vi "About.vi"(10 "窗口边界":T1) -> ()   [LabVIEW 2015]
doc: "本VI是为《我和LabVIEW》一书编写的示例。\n关于本书的介绍请参考网页：\nhttp://ruanqizhen.spaces.live.com/blog/cns!5852D4F797C53FB6!4310.entry"
uses:
  <vilib>/Utility/miscctls.llb/LVRectTypeDef.ctl
  user32.dll
panel:
  # "上海华湘计算机通讯工程有限公司\nShanghai Huaxiang \nCommunication Engineering Co.,Ltd.\n\nSwitch Matrix\nV1.0"
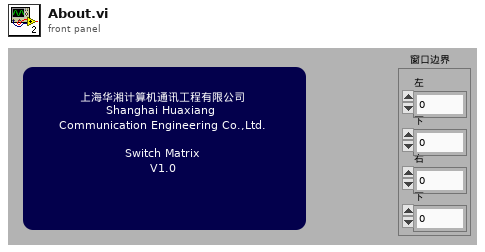
[diagram p1: front panel]
types:
  T1 = typedef "LVRectTypeDef.ctl" = cluster{"Left":i16, "Top":i16, "Right":i16, "Bottom":i16}
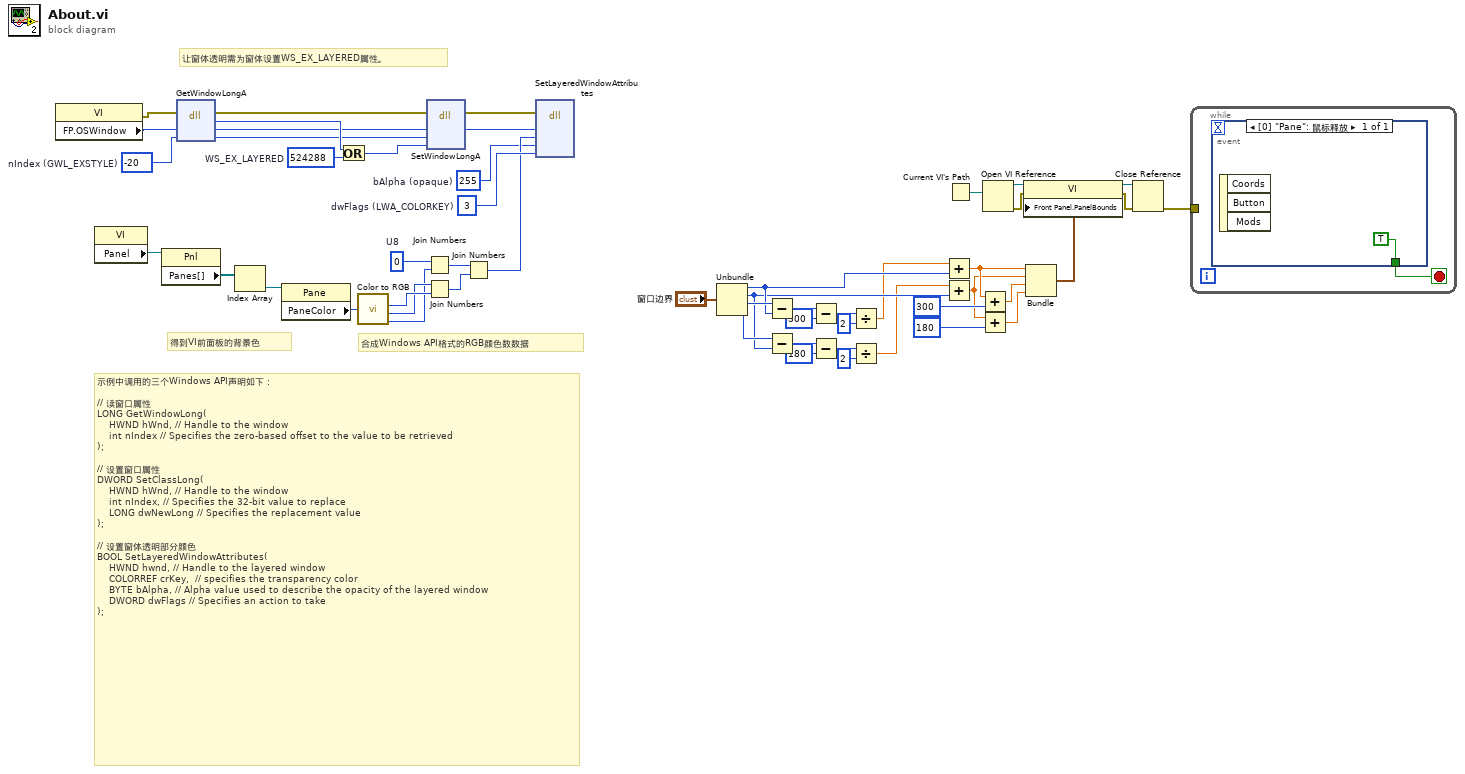
[diagram p0: block diagram]
diagram:
  w41 = 524288  # WS_EX_LAYERED
  w38 = -20  # nIndex (GWL_EXSTYLE)
  w44 = 255  # bAlpha (opaque)
  w45 = u8 0  # U8
  w49 = 3  # dwFlags (LWA_COLORKEY)
  # "示例中调用的三个Windows API声明如下：\n\n// 读窗口属性\nLONG GetWindowLong(      \n    HWND hWnd,\t// Handle to the window\n    int nIndex\t// Specifies the zero-based offset to the value to be retrieved\n);\n\n// 设置窗口属性\nDWORD SetClassLong(      \n    HWND hWnd,\t// Handle to the window\n    int nIndex,\t// Specifies the 32-bit value to replace\n    LONG dwNewLong // Specifies the replacement value\n);\n\n// 设置窗体透明部分颜色\nBOOL SetLayeredWindowAttributes(      \n    HWND hwnd,\t// Handle to the layered window\n    COLORREF crKey,  // specifies the transparency color\n    BYTE bAlpha,\t// Alpha value used to describe the opacity of the layered window\n    DWORD dwFlags\t// Specifies an action to take\n);"
  # "让窗体透明需为窗体设置WS_EX_LAYERED属性。"
  # "合成Windows API格式的RGB颜色数数据"
  # "得到VI前面板的背景色"
  n1 = property class="VI"() -> (error out=w36:errorcluster, "FP.OSWindow"=w40:i32)  [unwired: 2 in, 1 out]
  n2 = property class="VI"() -> ("Panel"=w52:refnum<vi>)  [unwired: 2 in, 2 out]
  n3 = property class="Pnl"(reference=w52) -> ("Panes[]"=w51:refnum<vi>[])  [unwired: 1 in, 2 out]
  n4 = dll-call lib="USER32.DLL" fn="GetWindowLongA" label="getWindowLong"(error in=w36, "handle"=w40, "nIndex"=w38) -> (error out=w35:errorcluster, w42:i32, "handle"=w39:i32, "nIndex"=w37:i32)  [unwired: 2 in, 1 out]
  n5 = Index Array(array=w51) -> (element=w50:refnum<vi>)  [unwired: 1 in]
  n6 = property class="Pane"(reference=w50) -> ("PaneColor"=w32:u32)  [unwired: 1 in, 2 out]
  n7 = Or(x=w42, y=w41) -> (x .or. y?=w43:i32)
  n8 = call <vilib>:"Color to RGB.vi"("Color"=w32) -> ("R"=w31:u8, "G"=w30:u8, "B"=w29:u8)  [unwired: 1 out]
  n9 = Join Numbers(hi=w45, lo=w29) -> ((hi.lo)=w47:u16)
  n10 = Join Numbers(hi=w30, lo=w31) -> ((hi.lo)=w48:u16)
  n11 = dll-call lib="USER32.DLL" fn="SetWindowLongA" label="SetWindowLong"(error in=w35, "handle"=w39, "nIndex"=w37, "dwNewLong"=w43) -> (error out=w34:errorcluster, "handle"=w33:i32)  [unwired: 4 in, 2 out]
  n12 = Join Numbers(hi=w47, lo=w48) -> ((hi.lo)=w46:u32)
  n13 = dll-call lib="USER32.DLL" fn="SetLayeredWindowAttributes" label="SetLayerdWindowAttributs"(error in=w34, "handle"=w33, "crkey"=w46, "bAlpha"=w44, "dwFlags"=w49) -> ()  [unwired: 6 in, 3 out]
  n14 = Unbundle("窗口边界") -> ("Left"=w13:i16, "Top"=w11:i16, "Right"=w14:i16, "Bottom"=w12:i16)
  n15 = Subtract(x=w14, y=w13) -> (x-y=w10:i16)
  n16 = Subtract(x=w12, y=w11) -> (x-y=w8:i16)
  n17 = Subtract(x=w10, y=i16 300) -> (x-y=w6:i16)
  n18 = Subtract(x=w8, y=i16 180) -> (x-y=w5:i16)
  n19 = Divide(x=w6, y=i16 2) -> (x/y=w2:dbl)
  n20 = Divide(x=w5, y=i16 2) -> (x/y=w1:dbl)
  n21 = Add(x=w2, y=w13) -> (x+y=w20:dbl)
  n22 = Add(x=w1, y=w11) -> (x+y=w19:dbl)
  n23 = Current VI's Path() -> (path=w28:path)
  n24 = Add(x=w20, y=i16 300) -> (x+y=w18:dbl)
  n25 = Add(x=w19, y=i16 180) -> (x+y=w17:dbl)
  n26 = Open VI Reference(vi path=w28) -> (vi reference=w27:refnum<vi>, error out=w26:errorcluster)  [unwired: 5 in]
  n27 = Bundle(w20, w19, w18, w17) -> (w16:cluster{dbl, dbl, dbl, dbl})  [unwired: 1 in]
  n28 = property class="VI"(reference=w27, error in=w26, "Front Panel.PanelBounds"=w16) -> (reference out=w24:refnum<vi>, error out=w25:errorcluster)
  n29 = Close Reference(reference=w24, error in (no error)=w25) -> (error out=w15:errorcluster)
  n30 = while {
    tunnel: w15 -> [_]
    stop <- w53 stop-if-true
    n31 = event shown="[0] \"Pane\": 鼠标释放" {
      selector: _ -> [_]
      dyn-events: _ -> [_]
      timeout: _ -> [_]
      tunnel: [TRUE] -> w53
      event Mouse Up {
        n32 = event-data() -> ()  [unwired: 4 out]
      }
    }
  }
